vi "VI cRIO Ueberwachung.vi"() -> (0 "error out":errorcluster)   [LabVIEW 2020, in "cRIO Ueberwachung.lvlib"]
uses:
  cRIO Ueberwachung.lvlib
  FGV Ausgaenge erzwingen Aktionen.ctl
  FGV Fehlerliste Aktionen.ctl
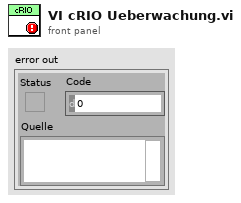
[diagram p1: front panel]
types:
  T1 = typedef "cRIO Ueberwachung.lvlib/FGV Fehlerliste Aktionen.ctl" = enum16{"lesen", "abfragen", "löschen", "laden", "speichern"}
  T2 = typedef "cRIO Ueberwachung.lvlib/FGV Ausgaenge erzwingen Aktionen.ctl" = enum16{"lesen", "starten", "erzwingen", "beenden"}
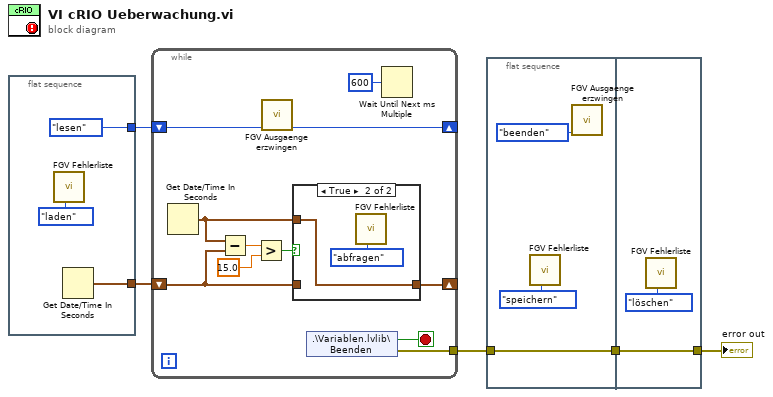
[diagram p0: block diagram]
diagram:
  n1 = flat-sequence {
    tunnel: [w8] -> w5
    tunnel: [FGV_Ausgaenge_erzwingen_Aktionen."lesen" ("Aktionen")] -> w4
    frame #0 {
      n2 = call "FGV Fehlerliste.vi"("Aktionen Fehlerliste"=FGV_Fehlerliste_Aktionen."laden") -> ()  [unwired: 9 in, 2 out]
      n3 = Get Date/Time In Seconds() -> (seconds since 1Jan1904=w8:timestamp)
    }
  }
  n4 = while {
    tunnel: [w14] -> w3
    shift-right: [w13] -> _
    shift-left: w5 -> [w11]
    shift-right: [w10] -> _
    shift-left: w4 -> [w9]
    stop <- w15 stop-if-true
    n5 = Get Date/Time In Seconds() -> (seconds since 1Jan1904=w12:timestamp)
    n6 = Subtract(x=w12, y=w11) -> (x-y=w18:dbl)
    n7 = Greater?(x=w18, y=15.0) -> (0:w16:bool)
    n8 = call "FGV Ausgaenge erzwingen.vi"("Aktionen"=w9) -> ("Aktionen"=w10:T2)  [unwired: 10 in]
    n9 = case shown="True" w16 {
      tunnel: w12 -> [_ w22]
      tunnel: w11 -> [w20 _]
      tunnel: [w20 w22] -> w13
      frame False {
      }
      frame True {
        n10 = call "FGV Fehlerliste.vi"("Aktionen Fehlerliste"=FGV_Fehlerliste_Aktionen."abfragen") -> ()  [unwired: 9 in, 2 out]
      }
    }
    n11 = shared-variable ".\\Variablen.lvlib\\Beenden"() -> (w15:bool, error out=w14:errorcluster)  [unwired: 1 in]
    n12 = Wait Until Next ms Multiple(millisecond multiple=u32 600 ("Vielfache von ms")) -> ()  [unwired: 1 out]
  }
  n13 = flat-sequence {
    tunnel: w3 -> [w25]
    tunnel: [w25] -> w1
    tunnel: [w27] -> w2
    tunnel: w1 -> [w27]
    frame #0 {
      n14 = call "FGV Fehlerliste.vi"("Aktionen Fehlerliste"=FGV_Fehlerliste_Aktionen."speichern") -> ()  [unwired: 9 in, 2 out]
      n15 = call "FGV Ausgaenge erzwingen.vi"("Aktionen"=FGV_Ausgaenge_erzwingen_Aktionen."beenden") -> ()  [unwired: 10 in, 1 out]
    }
    frame #1 {
      n16 = call "FGV Fehlerliste.vi"("Aktionen Fehlerliste"=FGV_Fehlerliste_Aktionen."löschen") -> ()  [unwired: 9 in, 2 out]
    }
  }
  "error out" <- w2
